vi "from string.vi"(8 "error in":errorcluster, 9 "data":string, 10 "version":string, 11 "Modbus Slave configuration in":refnum<class "Modbus Slave configuration.lvclass">) -> (0 "error out":errorcluster, 3 "Modbus Slave configuration out":refnum<class "Modbus Slave configuration.lvclass">)   [LabVIEW 2013, in "Modbus Slave configuration.lvclass"]
doc: "Provides an interface for loading a module configuration from a file or other serialized data source. It is recommended that all children of this class store data in two sets--data required for its own initialization, and any data required for parent initialization--and that each implementation uses the <b>Call Parent Method</b> primitive to de-serialize parent information. As a result, it is expected that every module configuration class calls <b>component configuration.lvclass:From String.vi</b>.Platypus Framework 1.0.1.65\nNI Systems Engineering - National Instruments"
uses:
  Modbus Slave configuration.lvclass
  module channel/Modbus Module Channel.lvclass
  <vilib>/NI/Tag Bus Module Framework/module configuration/TBM module configuration.lvclass
  Modbus Slave configuration.lvclass/Modbus Slave configuration.ctl
  <vilib>/NI/Tag Bus Module Framework/root configuration/TBM configuration.lvclass
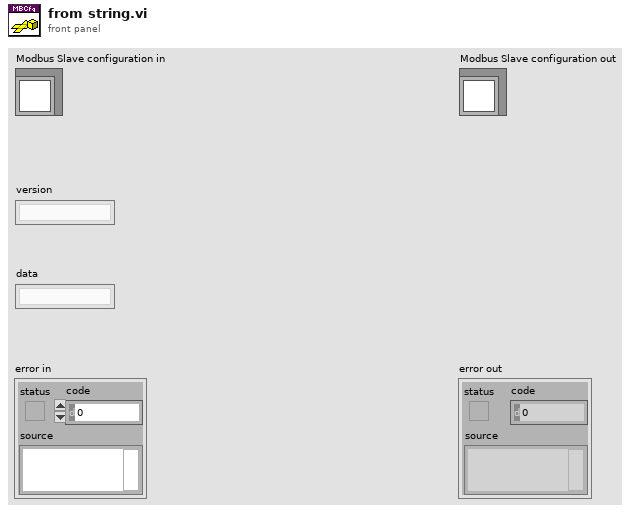
[diagram p1: front panel]
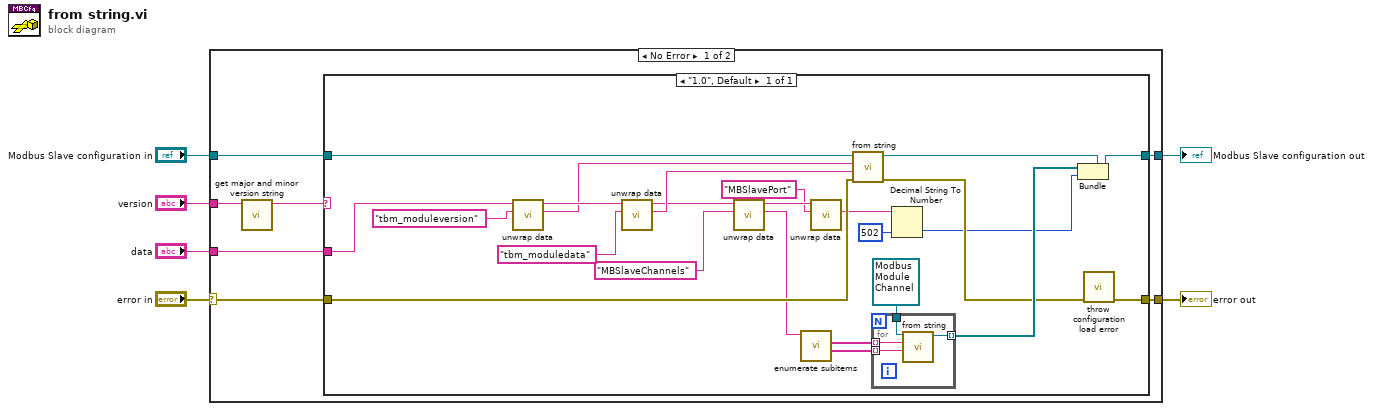
[diagram p0: block diagram]
diagram:
  n1 = case shown="No Error" "error in" {
    selector: "error in" -> [w7 w43]
    tunnel: "data" -> [w13 _]
    tunnel: "Modbus Slave configuration in" -> [w12 w42]
    tunnel: [w11 w42] -> w5
    tunnel: [w10 w43] -> w4
    tunnel: "version" -> [w9 _]
    frame No Error {
      n2 = call <vilib>:"get major and minor version string.vi"("full version"=w9) -> ("major.minor version"=w8:string)  [unwired: 10 in]
      n3 = case shown="\"1.0\", Default" w8 {
        tunnel: w13 -> [w33]
        tunnel: w7 -> [w32]
        tunnel: w12 -> [w37]
        tunnel: [w27] -> w11
        tunnel: [w35] -> w10
        frame "1.0", Default {
          n4 = call <vilib>:"unwrap data.vi"("identifier"="tbm_moduleversion" ("additional identifier"), "data to unwrap"=w33) -> ("unwrapped data"=w28:string, "remaining string"=w34:string)  [unwired: 8 in]
          n5 = call <vilib>:"unwrap data.vi"("identifier"="tbm_moduledata" ("additional identifier"), "data to unwrap"=w34) -> ("unwrapped data"=w30:string, "remaining string"=w26:string)  [unwired: 8 in]
          n6 = call <vilib>:"unwrap data.vi"("identifier"="MBSlaveChannels" ("additional identifier"), "data to unwrap"=w26) -> ("unwrapped data"=w24:string, "remaining string"=w19:string)  [unwired: 8 in]
          n7 = call <vilib>:"enumerate subitems.vi"("data to enumerate"=w24) -> ("associated data"=w22:string[], "discovered subitems"=w23:string[])  [unwired: 8 in, 1 out]
          n8 = call <vilib>:"unwrap data.vi"("identifier"="MBSlavePort" ("additional identifier"), "data to unwrap"=w19) -> ("unwrapped data"=w17:string)  [unwired: 8 in, 1 out]
          n9 = call-parent "from string.vi"("error in"=w32, "data"=w30, "version"=w28, "module configuration in"=w37) -> ("error out"=w20:errorcluster, "module configuration out"=w36:refnum<class "Modbus Slave configuration.lvclass">)  [unwired: 6 in]
          n10 = for {
            tunnel: w23 -> [w41] mode=indexing
            tunnel: w22 -> [w40] mode=indexing
            tunnel: [w39] -> w21 mode=indexing
            tunnel: refnum<class "Modbus Module Channel.lvclass"> refnum ("Modbus Module Channel.lvclass") -> [w38]
            n11 = call-dynamic "from string.vi"("channel data"=w40, "identifier"=w41, "channel in"=w38) -> ("channel out"=w39:refnum<class "Modbus Module Channel.lvclass">)  [unwired: 7 in, 1 out]
          }
          n12 = Decimal String To Number(string=w17, default (0L)=u16 502 ("default (0 I32)")) -> (number=w15:u16)  [unwired: 1 in, 1 out]
          n13 = Bundle(cluster=w36, w21, w15) -> (w27:refnum<class "Modbus Slave configuration.lvclass">)
          n14 = call <vilib>:"throw configuration load error.vi"("error in"=w20) -> ("error out"=w35:errorcluster)  [unwired: 10 in]
        }
      }
    }
    frame Error {
    }
  }
  "error out" <- w4
  "Modbus Slave configuration out" <- w5
